vi "BeepQueue.vi"(4 "error in":errorcluster, 6 "queueSize in (10)":i32=10, 7 "mode in (Get)":enum16{"Get", "Init", "Destroy"}(ring)) -> (0 "error out":errorcluster, 3 "queue out":refnum<queue>)   [LabVIEW 2010, in "Labricks.lvlib" / "Game.lvclass"]
uses:
  Game.lvclass
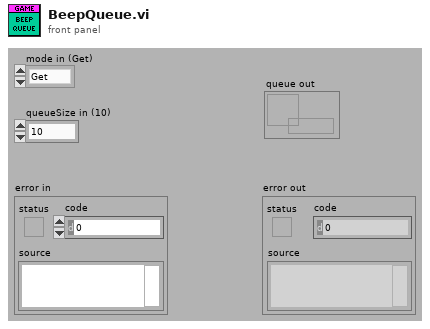
[diagram p1: front panel]
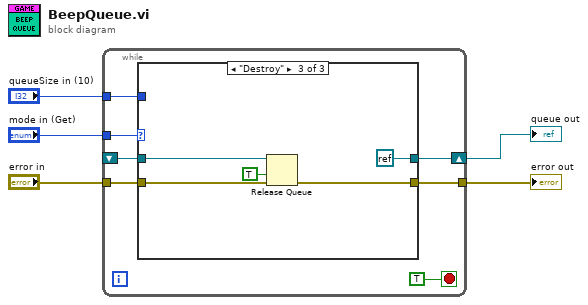
[diagram p0: block diagram]
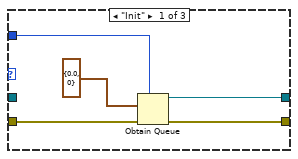
[diagram p2: hidden frame]
diagram:
  n1 = while {
    tunnel: "mode in (Get)" -> [w12]
    shift-right: [w11] -> w1
    shift-left: _ -> [w6]
    tunnel: "queueSize in (10)" -> [w10]
    tunnel: "error in" -> [w9]
    tunnel: [w8] -> w2
    stop <- TRUE stop-if-true
    n2 = case shown="\"Destroy\"" w12 {
      tunnel: [w16 w18 refnum<k0> refnum] -> w11
      tunnel: w10 -> [w15 _ _]
      tunnel: w9 -> [w14 w19 w24]
      tunnel: [w13 w19 w23] -> w8
      tunnel: w6 -> [_ w18 w22]
      frame "Init" {
        n3 = Obtain Queue(max queue size (-1, unlimited)=w15, element data type=cluster{"frequency":dbl, "duration":i32} {"frequency"=0.0, "duration"=0} ("BeepConfig"), error in (no error)=w14) -> (queue out=w16:refnum<queue>, error out=w13:errorcluster)  [unwired: 2 in, 1 out]
      }
      frame "Get" {
      }
      frame "Destroy" {
        n4 = Release Queue(queue=w22, force destroy? (F)=TRUE, error in (no error)=w24) -> (error out=w23:errorcluster)  [unwired: 2 out]
      }
    }
  }
  "queue out" <- w1
  "error out" <- w2
